vi "Undecimated Signal Decomposition and Reconstruction (UWT).vi"() -> ()   [LabVIEW 2023]
doc: "This example shows the undecimated wavelet transform-based signal decomposition and reconstruction with the WA Undecimated Wavelet Transform VI and the WA Inverse Undecimated Wavelet Transform VI. When the decomposition level increases, the approximation and the detail coefficients have coarse resolution. But the approximation and the detail coefficients at all levels have the same size as the input signal.\n\n<b>Instructions:</b>\n1) Run this VI.\n2) Observe results of the undecimated wavelet transform at different decomposition levels."
uses:
  <vilib>/addons/Wavelet Analysis/discrete wavelet transform.llb/WA 1D Undecimated Wavelet Transform (Waveform).vi
  <vilib>/addons/Wavelet Analysis/discrete wavelet transform.llb/WA Inverse 1D Undecimated Wavelet Transform (Waveform).vi
  <vilib>/addons/_Advanced Signal Processing/NI_AdvSigProcWA.lvlib
panel:
  in  "Data":u16(ring)=117 items=["1D Example Data"=100, "-"=101, "Doppler"=102, "HOP"=103, "TF Sine"=104, "Noisy Doppler"=105, "Sea Temperature"=106, "Sp500"=107, "Power Line"=108, "Engine Knocking"=109, "HeaviSine"=110, "Bumps"=111, "Blocks"=112, "Piece Regular"=113, "HypChirps"=114, "LinChirps"=115, "Chirps"=116, "Piece Polynomial"=117, "ECG"=131, "-"=118, "2D Example Data"=119, "-"=120, "Finger Print (Image)"=121, "Iris Flower (Image)"=122, "Mammogram (Image)"=123, "Lake (Image)"=127, "Two Can 1 (Image)"=132, "Two Can 2 (Image)"=133, "Camera Man (Image)"=134]
  in  "stop":bool
  out "Detail (level=3)":waveform(dbl)(graph)
  out "Detail (level=2)":waveform(dbl)(graph)
  out "Detail (level=1)":waveform(dbl)(graph)
  out "Approximation (level=3)":waveform(dbl)(graph)
  out "Reconstructed Signal":waveform(dbl)(graph)
  out "Signal":waveform(dbl)(graph)
  in  "Wavelet":u16(ring) items=["db02"=0, "db03"=1, "db04"=2, "db05"=3, "db06"=4, "db07"=5, "db08"=6, "db09"=7, "db10"=8, "db11"=9, "db12"=10, "db13"=11, "db14"=12, "Haar"=13, "bior1_3"=14, "bior1_5"=15, "bior2_2"=16, "bior2_4"=17, "bior2_6"=18, "bior2_8"=19, "bior3_1"=20, "bior3_3"=21, "bior3_5"=22, "bior3_7"=23, "bior3_9"=24, "bior4_4 (FBI)"=25, "bior5_5"=38, "bior6_8"=39, "coif1"=26, "coif2"=27, "coif3"=28, "coif4"=29, "coif5"=30, "sym2"=31, "sym3"=32, "sym4"=33, "sym5"=34, "sym6"=35, "sym7"=36, "sym8"=37]
  # "Overview: Shows the undecimated wavelet transform-based signal decomposition and reconstruction with the WA Undecimated Wavelet Transform VI and the WA Inverse Undecimated Wavelet Transform VI. \nRequirements: LabVIEW Full Development System, Advanced Signal Processing Toolkit\nInstructions: \n1. Run this VI.\n2. Observe results of the undecimated wavelet transform at different decomposition levels.\n3. Click Stop to stop the VI."
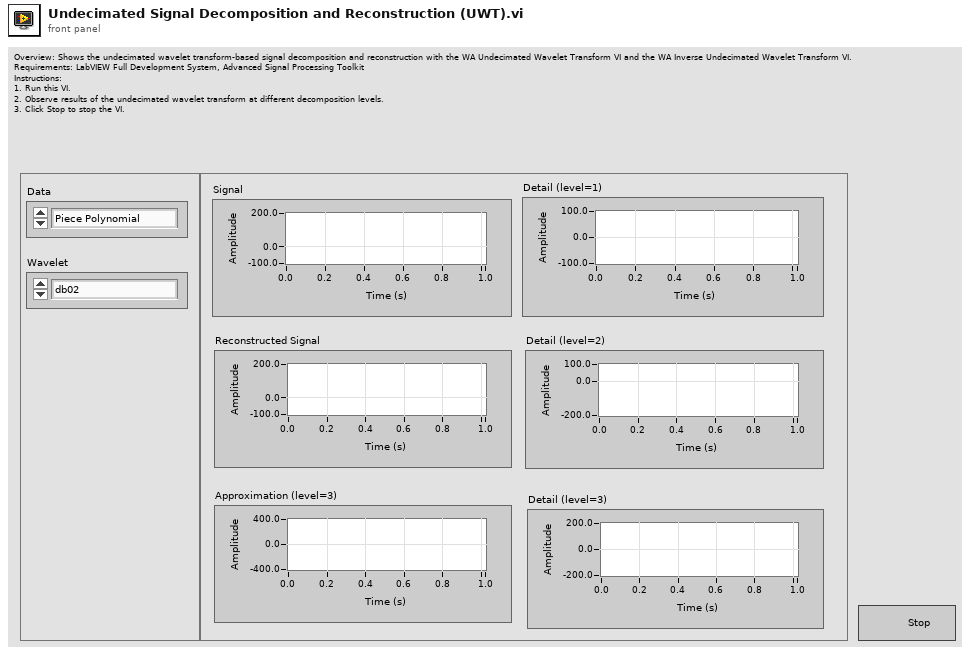
[diagram p1: front panel]
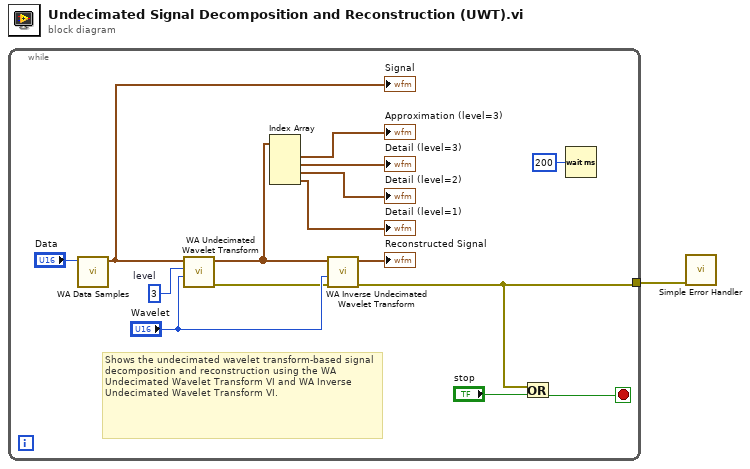
[diagram p0: block diagram]
diagram:
  n1 = while {
    tunnel: [w2] -> w1
    stop <- w5 stop-if-true
    w16 = 3  # level
    # "Shows the undecimated wavelet transform-based signal decomposition and reconstruction using the WA Undecimated Wavelet Transform VI and WA Inverse Undecimated Wavelet Transform VI."
    n2 = call <vilib>:"WA Data Samples.vi"("data"="Data") -> ("signal"=w14:waveform(dbl))  [unwired: 10 out]
    "Signal" <- w14
    n3 = call-poly <vilib>:"WA Undecimated Wavelet Transform.vi"("wavelet"="Wavelet", "levels"=w16, "signal"=w14) -> ("error out"=w7:errorcluster, "UWT coef"=w12:waveform(dbl)[])  [unwired: 1 in, 6 out]
    n4 = Index Array(array=w12) -> (element #1=→"Approximation (level=3)":waveform(dbl), element #2=→"Detail (level=3)":waveform(dbl), element #3=→"Detail (level=2)":waveform(dbl), element #4=→"Detail (level=1)":waveform(dbl))  [unwired: 4 in]
    n5 = call-poly <vilib>:"WA Inverse Undecimated Wavelet Transform.vi"("error in (no error)"=w7, "wavelet"="Wavelet", "UWT coef"=w12) -> ("error out"=w2:errorcluster, "signal"=→"Reconstructed Signal":waveform(dbl))  [unwired: 7 out]
    n6 = Or(x=w2, y="stop") -> (x .or. y?=w5:bool)
    n7 = Wait (ms)(milliseconds to wait=u32 200 ("millisecond multiple")) -> ()  [unwired: 1 out]
  }
  n8 = call <vilib>:"Simple Error Handler.vi"("error in (no error)"=w1) -> ()  [unwired: 1 in, 8 out]
